vi "Logger-Flush Log.vi"(0 "State in":T1) -> (4 "State out":T1, 15 "error out":errorcluster)   [LabVIEW 2020]
uses:
  Typedefs/Logger-State.ctl
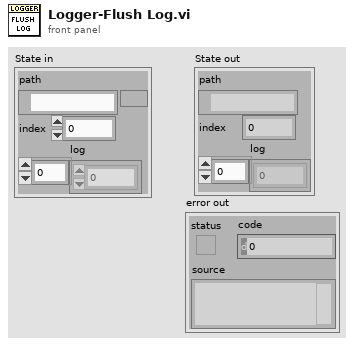
[diagram p1: front panel]
types:
  T1 = typedef "Logger-State.ctl" = cluster{"path":path, "index":i32, "log":u8[]}
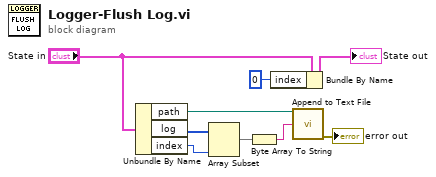
[diagram p0: block diagram]
diagram:
  n1 = Unbundle By Name("State in") -> ("path"=w7:path, "log"=w6:u8[], "index"=w5:i32)
  n2 = Array Subset(array=w6, length=w5) -> (w4:u8[])  [unwired: 1 in]
  n3 = Byte Array To String(unsigned byte array=w4) -> (string=w3:string)
  n4 = Bundle By Name(cluster="State in", "index"=0) -> (→"State out":T1)
  n5 = call "Append to Text File.vi"("file path"=w7, "text"=w3) -> ("error out"=→"error out":errorcluster)  [unwired: 12 in, 1 out]
